vi "Fields Get For Sequence.vi"(8 "error in (no error)":errorcluster, 10 "sxSequenceId (\"\")":string, 11 "Connection Refnum":T1) -> (0 "error out":errorcluster, 1 "Current Sequence Fields":T2[](array[typedef]), 2 "All Custom Fields":T2[](array[typedef]), 3 "Connection Refnum":T1)   [LabVIEW 2011]
uses:
  Field Record.ctl
  Field DataTypes.ctl
  Field NextItem.ctl
  Summitek EXT/ODBC/SQL Controls/Connection Refnum.ctl
  Field Order By.ctl
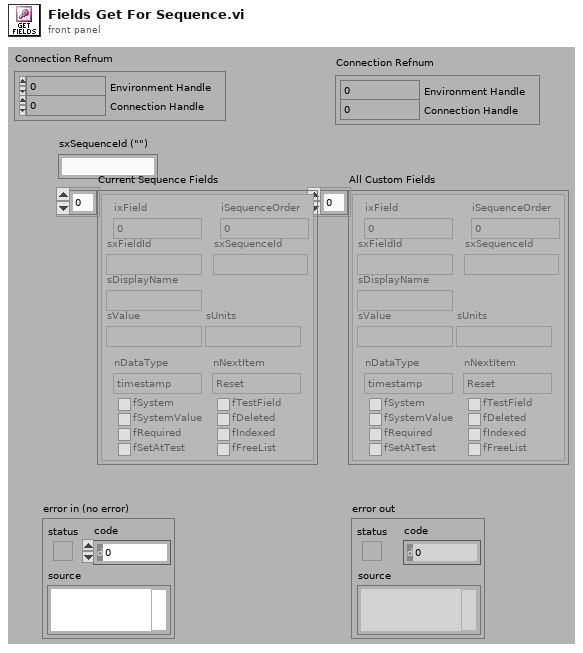
[diagram p1: front panel]
types:
  T1 = typedef "Connection Refnum.ctl" = cluster{"Environment Handle":i32, "Connection Handle":i32}
  T2 = typedef "Field Record.ctl" = cluster{"ixField":i32, "iSequenceOrder":i32, "sxFieldId":string, "sxSequenceId":string, "sDisplayName":string, "sValue":string, "sUnits":string, "nDataType":T3, "nNextItem":T4, "fSystem":bool, "fSystemValue":bool, "fRequired":bool, "fSetAtTest":bool, "fTestField":bool, "fDeleted":bool, "fIndexed":bool, "fFreeList":bool}
  T3 = typedef "Field DataTypes.ctl" = enum32{"text", "numeric", "list", "timestamp", "boolean"}
  T4 = typedef "Field NextItem.ctl" = enum32{"Reset", "Retain", "Auto-Increment"}
  T5 = typedef "Field Order By.ctl" = enum32{"sxSequenceId", "sxFieldId", "sDisplayName", "sValue", "fSetAtTest", "fRequired", "nNextItem"}
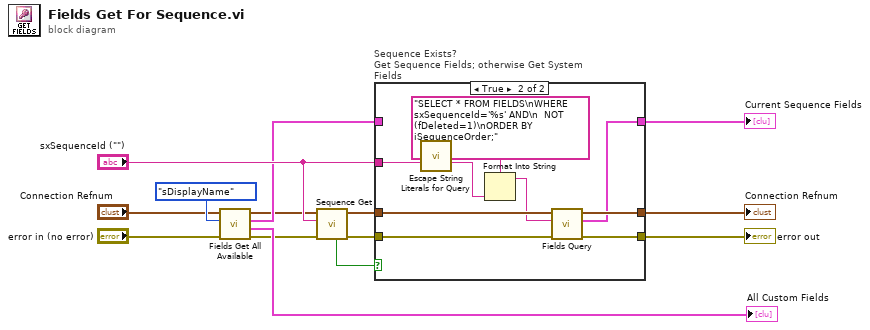
[diagram p0: block diagram]
diagram:
  n1 = call "Fields Get All Available.vi"("error in (no error)"="error in (no error)", "Sort by (sxSequenceId)"=Field_Order_By."sDisplayName", "Connection Refnum"="Connection Refnum") -> ("error out"=w6:errorcluster, "Custom Fields"=→"All Custom Fields":T2[], "System or ALL Combined Fields"=w9:T2[], "Connection Refnum"=w8:T1)  [unwired: 2 in, 3 out]
  n2 = call "Sequence Get.vi"("error in (no error)"=w6, "sxSequenceId (\"\")"="sxSequenceId (\"\")", "Connection Refnum"=w8) -> ("error out"=w5:errorcluster, "Connection Refnum"=w7:T1, "Data Present"=w12:bool)  [unwired: 6 out]
  n3 = case "Sequence Exists?\nGet Sequence Fields; otherwise Get System Fields" shown="True" w12 {
    tunnel: w5 -> [w16 w21]
    tunnel: [w17 w18] -> w14
    tunnel: w7 -> [w15 w23]
    tunnel: [w16 w20] -> w1
    tunnel: [w15 w22] -> w2
    tunnel: "sxSequenceId (\"\")" -> [_ w24]
    tunnel: w9 -> [w17 _]
    frame False {
    }
    frame True {
      n4 = call "Escape String Literals for Query.vi"("String"=w24) -> ("escaped String"=w26:string)  [unwired: 1 in, 13 out]
      n5 = Format Into String(format string="SELECT * FROM FIELDS\nWHERE sxSequenceId='%s' AND\n  NOT (fDeleted=1)\nORDER BY iSequenceOrder;" ("User Query"), w26) -> (resulting string=w19:string)  [unwired: 2 in, 1 out]
      n6 = call "Fields Query.vi"("error in (no error)"=w21, "Query"=w19, "Connection Refnum"=w23) -> ("error out"=w20:errorcluster, "Fields"=w18:T2[], "Connection Refnum"=w22:T1)  [unwired: 1 in, 5 out]
    }
  }
  "error out" <- w1
  "Current Sequence Fields" <- w14
  "Connection Refnum" <- w2
